vi "Send CONNACK.vi"(8 "error in (no error)":errorcluster, 10 "Conn Return Code":T1=enum."Connection refused: not authorized", 11 "connection ID":refnum<k5>) -> (0 "error out":errorcluster, 2 "ConnAck Message":u8[](array[numeric]) format="%x", 3 "connection ID out":refnum<k5>)   [LabVIEW 2020, in "DAQIO MQTT.lvlib"]
uses:
  DAQIO MQTT.lvlib
  Controls/MessageType.ctl
  Controls/Connection Return Codes.ctl
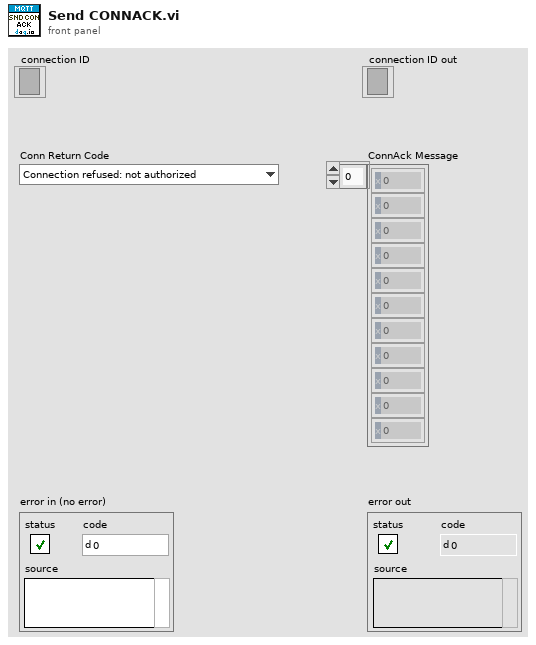
[diagram p1: front panel]
types:
  T1 = typedef "DAQIO MQTT.lvlib/Connection Return Codes.ctl" = enum16{"Connection accepted", "Connection refused: unacceptable protocol version", "Connection refused: identifier rejected", "Connection refused: Server unavailable", "Connection refused: bad user name or password", "Connection refused: not authorized"}
  T2 = typedef "DAQIO MQTT.lvlib/MessageType.ctl" = enum32{"Reserved", "CONNECT", "CONNACK", "PUBLISH", "PUBACK", "PUBREC", "PUBREL", "PUBCOMP", "SUBSCRIBE", "SUBACK", "UNSUBSCRIBE", "UNSUBACK", "PINGREQ", "PINGRESP", "DISCONNECT", "Reserved2"}
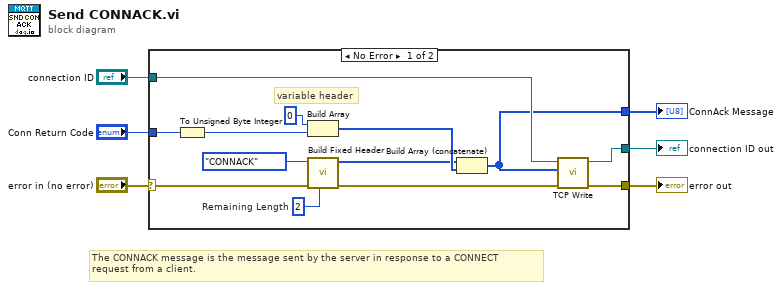
[diagram p0: block diagram]
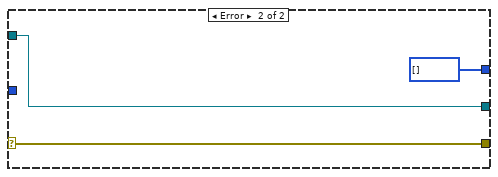
[diagram p2: hidden frame]
diagram:
  # "The CONNACK message is the message sent by the server in response to a CONNECT\nrequest from a client."
  n1 = case shown="No Error" "error in (no error)" {
    selector: "error in (no error)" -> [w15 w22]
    tunnel: [w11 w22] -> w5
    tunnel: "Conn Return Code" -> [w10 _]
    tunnel: "connection ID" -> [w9 w21]
    tunnel: [w8 w21] -> w2
    tunnel: [w7 u8[] []] -> w1
    frame No Error {
      w16 = u32 2  # Remaining Length
      # "variable header"
      n2 = To Unsigned Byte Integer(number=w10) -> (unsigned 8bit integer=w13:u8)
      n3 = Build Array(u8 0 ("element"), w13) -> (w19:u8[])
      n4 = call "Build Fixed Header.vi"("Remaining Length"=w16, "error in (no error)"=w15, "MessageType"=MessageType."CONNACK") -> ("error out"=w12:errorcluster, "Fixed Header"=w17:u8[])  [unwired: 7 in]
      n5 = Build Array (concatenate)(w17, w19) -> (w7:u8[])
      n6 = call "TCP Write.vi"("error in (no error)"=w12, "data in"=w7, "connection ID"=w9) -> ("error out"=w11:errorcluster, "connection ID out"=w8:refnum<k5>)  [unwired: 6 in, 1 out]
    }
    frame Error {
    }
  }
  "error out" <- w5
  "connection ID out" <- w2
  "ConnAck Message" <- w1
